vi "inclineDisplay.vi"(0 "refnum in":refnum<file>, 1 "inclineMin":dbl=20.0, 2 "inclineMid":dbl=40.0, 3 "inclineMax":dbl=78.0, 5 "VISA resource name":refnum<visa-resource-name>, 7 "write buffer":string="G\u0002", 9 "E-Stop/Incline":bool, 11 "error in":errorcluster) -> (4 "INCLINE":dbl(graph), 6 "resultIncline":bool, 15 "error out":errorcluster)   [LabVIEW 2018]
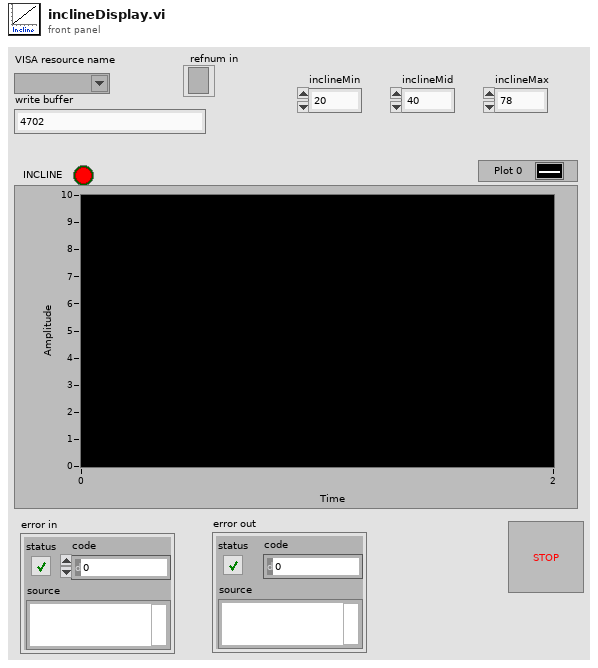
[diagram p1: front panel]
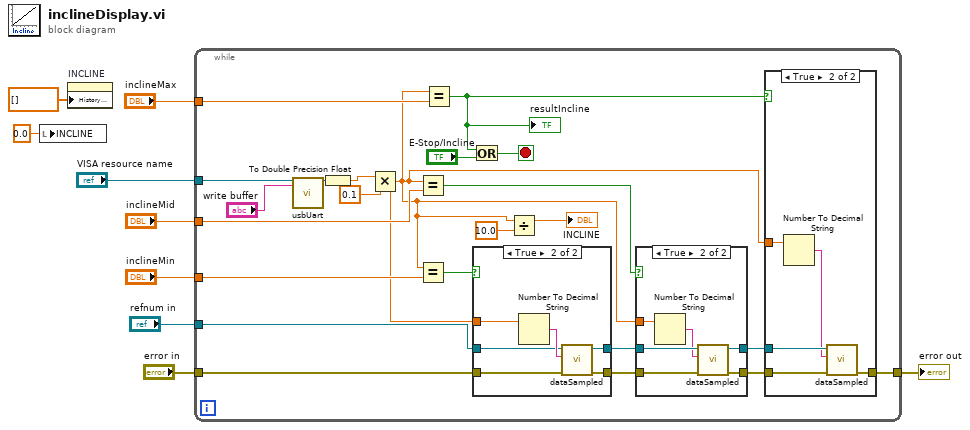
[diagram p0: block diagram]
diagram:
  n1 = local write "INCLINE"(0.0 ("INCLINE")) -> ()
  n2 = property on="INCLINE" class="WFChart (strict)"("History Data"=dbl[] []) -> ()  [unwired: 2 in, 2 out]
  n3 = while {
    tunnel: "error in" -> [w31]
    tunnel: [w20] -> w7
    tunnel: "refnum in" -> [w19]
    tunnel: "inclineMin" -> [w18]
    tunnel: "inclineMid" -> [w17]
    tunnel: "inclineMax" -> [w16]
    tunnel: "VISA resource name" -> [w15]
    stop <- w23 stop-if-true
    n4 = call "usbUart.vi"("VISA resource name"=w15, "write buffer"="write buffer") -> ("number[0]"=w24:u32)  [unwired: 6 in, 11 out]
    n5 = To Double Precision Float(number=w24) -> (double precision float=w11:dbl)
    n6 = Multiply(x=w11, y=0.1) -> (x*y=w12:dbl)
    n7 = Equal?(x=w12, y=w17) -> (x = y?=w25:bool)
    n8 = Equal?(x=w12, y=w18) -> (x = y?=w30:bool)
    n9 = Equal?(x=w12, y=w16) -> (x = y?=w21:bool)
    "resultIncline" <- w21
    n10 = Or(x=w21, y="E-Stop/Incline") -> (x .or. y?=w23:bool)
    n11 = case shown="True" w30 {
      tunnel: w31 -> [w48 w54]
      tunnel: w12 -> [_ w52]
      tunnel: [w47 w51] -> w29
      tunnel: [w48 w50] -> w28
      tunnel: w19 -> [w47 w49]
      frame False {
      }
      frame True {
        n12 = Number To Decimal String(number=w52) -> (decimal integer string=w53:string)  [unwired: 1 in]
        n13 = call "dataSampled.vi"("Error In"=w54, "Data"=w53, "refnum in"=w49) -> ("error out"=w50:errorcluster, "refnum out"=w51:refnum<file>)  [unwired: 7 in]
      }
    }
    n14 = Divide(x=w12, y=10.0) -> (x/y=→"INCLINE":dbl)
    n15 = case shown="True" w25 {
      tunnel: w29 -> [w40 w46]
      tunnel: w28 -> [w39 w45]
      tunnel: w12 -> [_ w43]
      tunnel: [w40 w42] -> w27
      tunnel: [w39 w41] -> w26
      frame False {
      }
      frame True {
        n16 = Number To Decimal String(number=w43) -> (decimal integer string=w44:string)  [unwired: 1 in]
        n17 = call "dataSampled.vi"("Error In"=w45, "Data"=w44, "refnum in"=w46) -> ("error out"=w41:errorcluster, "refnum out"=w42:refnum<file>)  [unwired: 7 in]
      }
    }
    n18 = case shown="True" w21 {
      tunnel: w27 -> [_ w38]
      tunnel: w26 -> [w33 w37]
      tunnel: w12 -> [_ w35]
      tunnel: [w33 w34] -> w20
      frame False {
      }
      frame True {
        n19 = Number To Decimal String(number=w35) -> (decimal integer string=w36:string)  [unwired: 1 in]
        n20 = call "dataSampled.vi"("Error In"=w37, "Data"=w36, "refnum in"=w38) -> ("error out"=w34:errorcluster)  [unwired: 7 in, 1 out]
      }
    }
  }
  "error out" <- w7
